vi "get_reference_data.vi"(7 "active_reference_name":string, 8 "error_in":errorcluster, 11 "all_config_info":T1 {"main_ini_file"."SCANNER Flow control" items=["None"=0, "XON/XOFF"=1, "RTS/CTS"=2, "DTR/DSR"=4]; "main_ini_file"."SCANNER Stop bits" items=["1.0"=10, "1.5"=15, "2.0"=20]}) -> (0 "error_out":errorcluster)   [LabVIEW 2019]
uses:
  ini/typedef/DOCK_all_config_info.ctl
  ini/typedef/DOCK_main_ini_file.ctl
  queues/typedef/DOCK_queue_refnums.ctl
  queues/typedef/DOCK_MAIN_queue_element.ctl
  DOCK_MAIN_sequence_state.ctl
  queues/typedef/DOCK_SCANNER_queue_element.ctl
  SCANNER/DOCK_SCANNER_sequence_state.ctl
  queues/typedef/DOCK_PRINTER_queue_element.ctl
  PRINTER/DOCK_PRINTER_sequence_state.ctl
  FGV/SQL_connection/FGV_DOCK_SQL_connection.ctl
  FGV/DOCK_records_display/FGV_DOCK_records_display.ctl
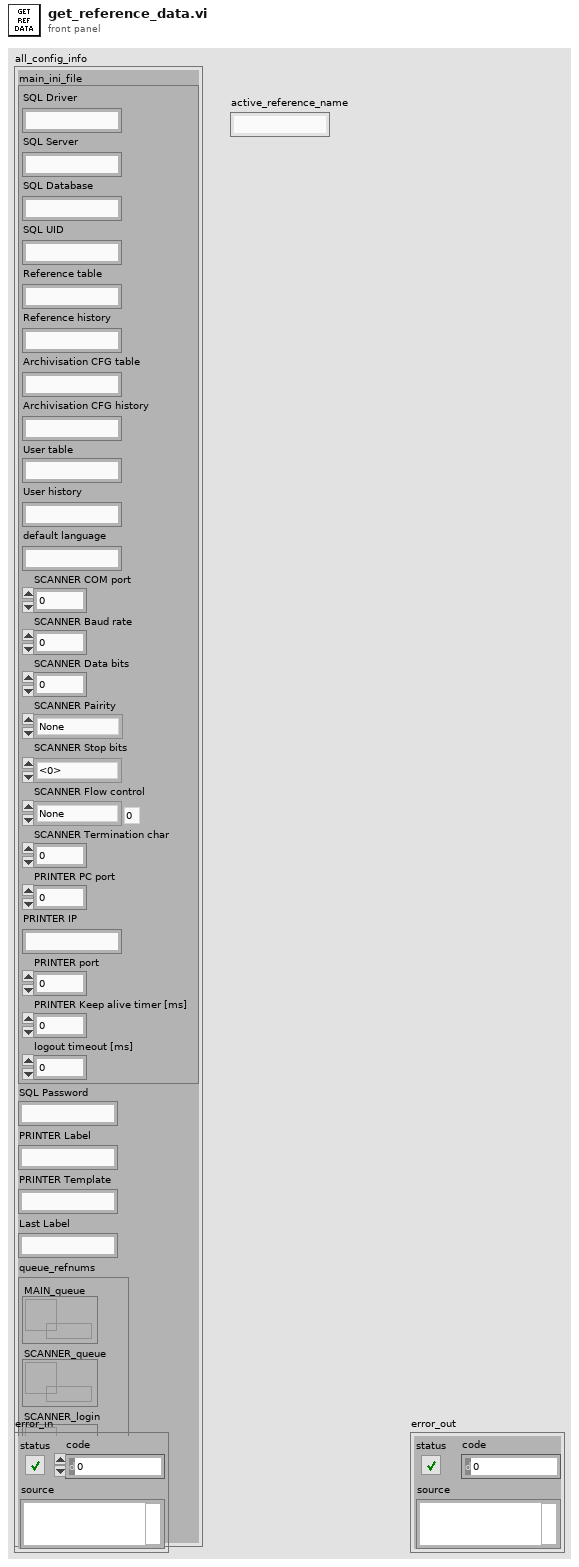
[diagram p1: front panel]
types:
  T1 = typedef "DOCK_all_config_info.ctl" = cluster{"main_ini_file":T2, "SQL Password":string, "PRINTER Label":string, "PRINTER Template":string, "Last Label":string, "queue_refnums":T3}
  T2 = typedef "DOCK_main_ini_file.ctl" = cluster{"SQL Driver":string, "SQL Server":string, "SQL Database":string, "SQL UID":string, "Reference table":string, "Reference history":string, "Archivisation CFG table":string, "Archivisation CFG history":string, "User table":string, "User history":string, "default language":string, "SCANNER COM port":u16, "SCANNER Baud rate":u32, "SCANNER Data bits":u16, "SCANNER Pairity":enum16{"None", "Odd", "Even", "Mark", "Space"}, "SCANNER Stop bits":u16, "SCANNER Flow control":u16, "SCANNER Termination char":u8, "PRINTER PC port":u16, "PRINTER IP":string, "PRINTER port":u16, "PRINTER Keep alive timer [ms]":i32, "logout timeout [ms]":i32}
  T3 = typedef "DOCK_queue_refnums.ctl" = cluster{"MAIN_queue":refnum<queue>, "SCANNER_queue":refnum<queue>, "SCANNER_login":refnum<queue>, "PRINTER_queue":refnum<queue>}
  T4 = typedef "FGV_DOCK_records_display.ctl" = enum16{"initialize", "set_reference_data", "set_serial", "set_header", "set_operations", "set_results", "set_batches", "get_reference_data", "get_part_number_ref", "get_serial", "get_batch_code", "get_gear_ID", "get_operation_IDs", "toggle_results", "show_all_results", "hide_all_results", "display", "clear"}
  T5 = typedef "FGV_DOCK_SQL_connection.ctl" = enum16{"initialize", "connect", "read_tables", "read_columns", "SELECT", "INSERT", "UPDATE", "DELETE", "EXEC + headers", "EXEC", "TRANSACTION", "connection_active?", "disconnect"}
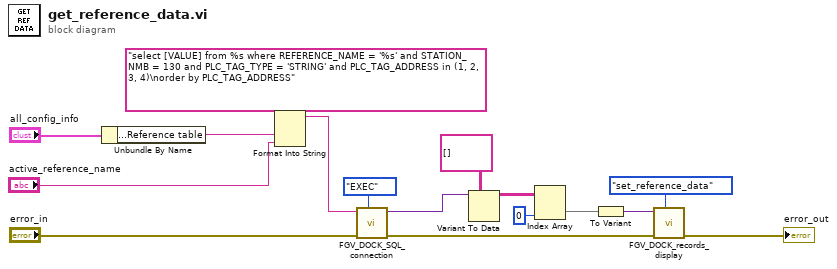
[diagram p0: block diagram]
diagram:
  n1 = Unbundle By Name("all_config_info") -> ("main_ini_file.Reference table"=w7:string)
  n2 = Format Into String(format string="select [VALUE] from %s where REFERENCE_NAME = '%s' and STATION_NMB = 130 and PLC_TAG_TYPE = 'STRING' and PLC_TAG_ADDRESS in (1, 2, 3, 4)\norder by PLC_TAG_ADDRESS" ("SQL_statement"), w7, "active_reference_name") -> (resulting string=w6:string)  [unwired: 2 in, 1 out]
  n3 = call "FGV_DOCK_SQL_connection.vi"("options"=FGV_DOCK_SQL_connection."EXEC", "error_in"="error_in", "SQL_statement"=w6) -> ("error_out"=w8:errorcluster, "SQL_result"=w13:variant)  [unwired: 4 in, 3 out]
  n4 = Variant To Data(type=string[][] [], Variant=w13) -> (data=w11:string[][])  [unwired: 1 in, 1 out]
  n5 = Index Array(array=w11, index (col)=0 ("disabled index (col)")) -> (element=w15:string[])  [unwired: 1 in]
  n6 = To Variant(anything=w15) -> (Variant=w16:variant)
  n7 = call "FGV_DOCK_records_display.vi"("options"=FGV_DOCK_records_display."set_reference_data", "error_in"=w8, "input"=w16) -> ("error_out"=→"error_out":errorcluster)  [unwired: 7 in, 1 out]
